vi "rad_Check IF 903x.vi"(11 "Product Name":string) -> (3 "Found 903x?":bool)   [LabVIEW 2015]
panel:
  out "Model":string
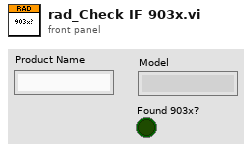
[diagram p1: front panel]
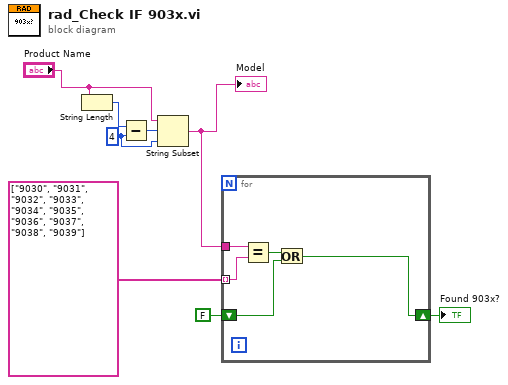
[diagram p0: block diagram]
diagram:
  w6 = 4 ("y")
  n1 = String Length(string="Product Name") -> (length=w7:i32)
  n2 = Subtract(x=w7, y=w6) -> (x-y=w8:i32)
  n3 = String Subset(string="Product Name", offset (0)=w8, length (rest)=w6) -> (substring=w3:string)
  "Model" <- w3
  n4 = for {
    tunnel: string[] ["9030", "9031", "9032", "9033", "9034", "9035", "9036", "9037", "9038", "9039"] -> [w12] mode=indexing
    tunnel: w3 -> [w13]
    shift-right: [w9] -> w1
    shift-left: FALSE -> [w10]
    n5 = Equal?(x=w13, y=w12) -> (x = y?=w11:bool)
    n6 = Or(x=w11, y=w10) -> (x .or. y?=w9:bool)
  }
  "Found 903x?" <- w1
